vi "例7-3(1).vi"() -> ()   [LabVIEW 2019]
uses:
  <vilib>/measure/NI_MABase.lvlib
panel:
  in  "端口":u16=6040
  in  "停止按钮":bool
  out "波形图（服务器）":waveform(dbl)(graph)
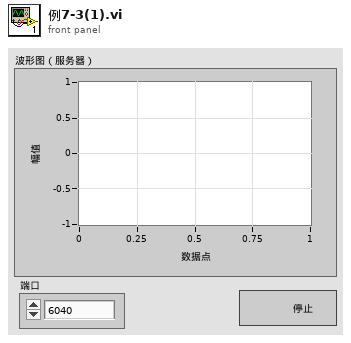
[diagram p1: front panel]
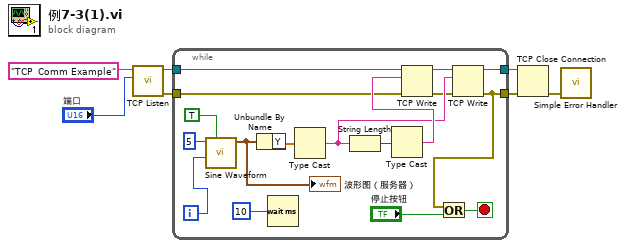
[diagram p0: block diagram]
diagram:
  n1 = call <vilib>:"TCP Listen.vi"("port"="端口", "service name"="TCP  Comm Example") -> ("error out"=w3:errorcluster, "connection ID"=w5:refnum<k5>)  [unwired: 5 in, 3 out]
  n2 = while {
    tunnel: w5 -> [w21]
    tunnel: [w19] -> w4
    tunnel: w3 -> [w18]
    tunnel: [w16] -> w2
    i -> [w10]
    stop <- w14 stop-if-true
    n3 = call <vilib>:"Sine Waveform.vi"("reset signal"=TRUE, "phase"=w10, "frequency"=5 ("samples")) -> ("signal out"=w9:waveform(dbl))  [unwired: 7 in, 1 out]
    "波形图（服务器）" <- w9
    n4 = Unbundle By Name(w9) -> ("Y"=w11:dbl[])
    n5 = Wait (ms)(milliseconds to wait=10) -> ()  [unwired: 1 out]
    n6 = Type Cast(x=w11) -> (*(type *) &x=w22:string)  [unwired: 1 in]
    n7 = String Length(string=w22) -> (length=w24:i32)
    n8 = Type Cast(x=w24) -> (*(type *) &x=w23:string)  [unwired: 1 in]
    n9 = TCP Write(connection ID=w21, data in=w23, error in (no error)=w18) -> (connection ID out=w20:refnum<k5>, error out=w17:errorcluster)  [unwired: 1 in, 1 out]
    n10 = TCP Write(connection ID=w20, data in=w22, error in (no error)=w17) -> (connection ID out=w19:refnum<k5>, error out=w16:errorcluster)  [unwired: 1 in, 1 out]
    n11 = Or(x=w16, y="停止按钮") -> (x .or. y?=w14:bool)
  }
  n12 = TCP Close Connection(connection ID=w4, error in (no error)=w2) -> (error out=w1:errorcluster)  [unwired: 1 in, 1 out]
  n13 = call <vilib>:"Simple Error Handler.vi"("error in (no error)"=w1) -> ()  [unwired: 4 in, 5 out]
